vi "Write Variable (multirow).vi"(6 "Time Stamps":timestamp[](array[timestamp]), 8 "error in (no error)":errorcluster, 9 "Data":variant, 10 "variable":string, 11 "Data.PG in":refnum<class "LV-Data.PGSQL.lvclass">) -> (0 "error out":errorcluster, 1 "Wrote to DB?":bool, 2 "Paths out":string, 3 "Data.PG out":refnum<class "LV-Data.PGSQL.lvclass">)   [LabVIEW 2019, in "LV-Data.PGSQL.lvclass"]
uses:
  LV-Data.PGSQL.lvclass
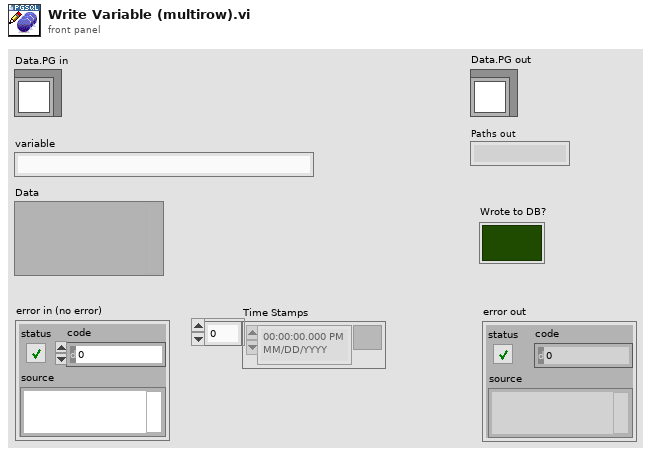
[diagram p1: front panel]
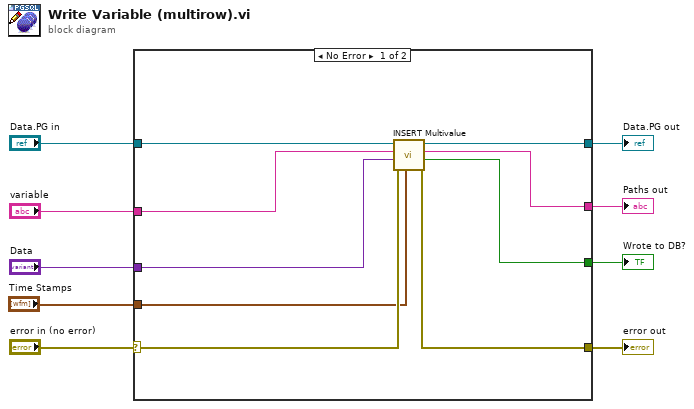
[diagram p0: block diagram]
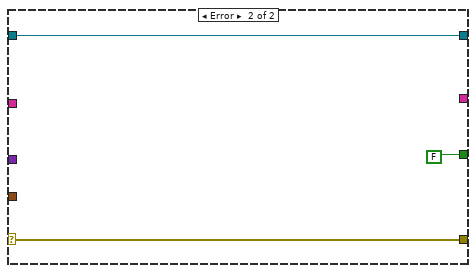
[diagram p2: hidden frame]
diagram:
  n1 = case shown="No Error" "error in (no error)" {
    selector: "error in (no error)" -> [w14 w21]
    tunnel: "Data.PG in" -> [w18 w20]
    tunnel: [w13 _] -> w1
    tunnel: "variable" -> [w17 _]
    tunnel: "Data" -> [w16 _]
    tunnel: [w15 w20] -> w6
    tunnel: [w12 w21] -> w4
    tunnel: "Time Stamps" -> [w11 _]
    tunnel: [w10 FALSE ("Wrote to DB?")] -> w2
    frame No Error {
      n2 = call "INSERT Multivalue.vi"("Array"=w11, "error in"=w14, "Data"=w16, "Path(s)"=w17, "Data.PG in"=w18) -> ("error out"=w12:errorcluster, "Wrote to DB?"=w10:bool, "Paths out"=w13:string, "Data.PG out"=w15:refnum<class "LV-Data.PGSQL.lvclass">)  [unwired: 3 in]
    }
    frame Error {
    }
  }
  "Wrote to DB?" <- w2
  "Data.PG out" <- w6
  "error out" <- w4
  "Paths out" <- w1
